vi "time_count_insert_in_table.vi"(8 "error in (no error)":errorcluster, 10 "time in sec":dbl[](array[numeric]), 11 "bd count array":dbl[](array[numeric])) -> (0 "error out":errorcluster, 3 "Array 3":dbl[][](array[numeric]))   [LabVIEW 2017]
panel:
  out "deleted portion":dbl[](array[numeric])
  out "array w/ subset deleted":dbl[](array[numeric])
  out "element":dbl
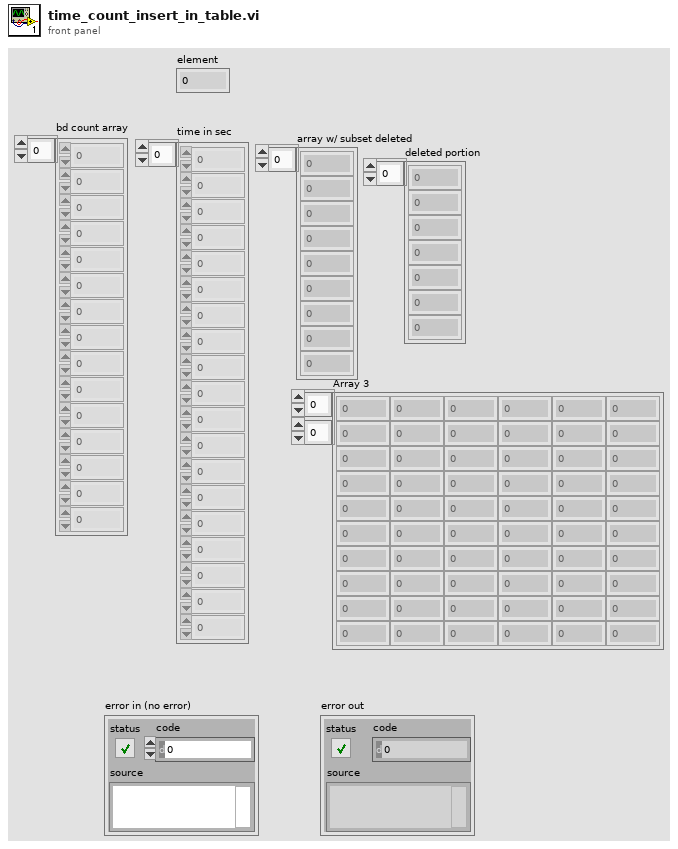
[diagram p1: front panel]
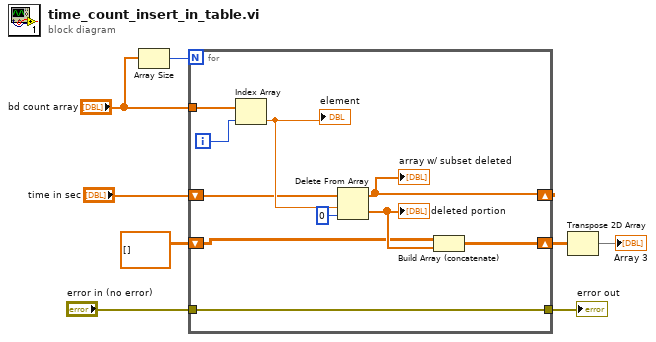
[diagram p0: block diagram]
diagram:
  n1 = Array Size(array="bd count array") -> (size(s)=w8:i32)
  n2 = for {
    N: w8 -> [_]
    tunnel: "bd count array" -> [w18]
    shift-right: [w14] -> _
    shift-left: "time in sec" -> [w13]
    shift-right: [w12] -> w4
    shift-left: dbl[][] [] -> [w10]
    tunnel: [w9] -> w2
    tunnel: "error in (no error)" -> [w9]
    i -> [w16]
    n3 = Index Array(array=w18, index=w16) -> (element=w17:dbl)
    "element" <- w17
    n4 = Delete From Array(array=w13, length=w17, index=0) -> (deleted portion=w11:dbl[], array with subset deleted=w14:dbl[])
    "array w/ subset deleted" <- w14
    "deleted portion" <- w11
    n5 = Build Array (concatenate)(w10, w11) -> (w12:dbl[][])
  }
  "error out" <- w2
  n6 = Transpose 2D Array(2D array=w4) -> (transposed array=→"Array 3":dbl[][])
